vi "Dimmer FG.vi"(7 "Operation":enum16{"Init", "Run", "Close Ref"}(ring)=enum."Run", 8 "error in":errorcluster, 10 "dimmer":i8) -> (0 "error out":errorcluster)   [LabVIEW 2013]
uses:
  System.Management
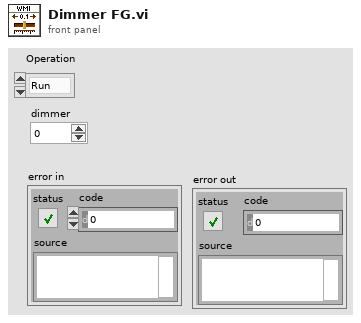
[diagram p1: front panel]
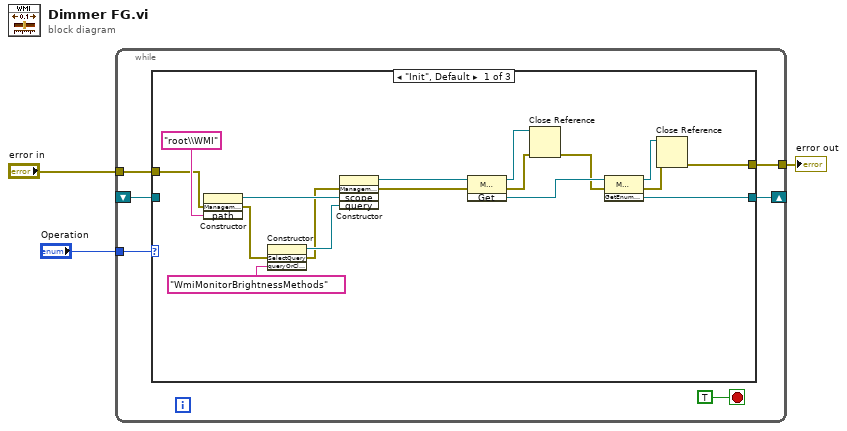
[diagram p0: block diagram]
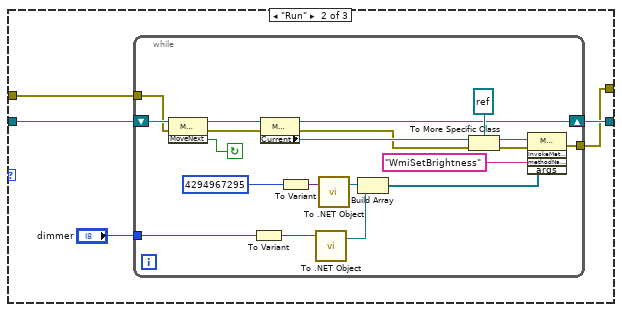
[diagram p2: hidden frame]
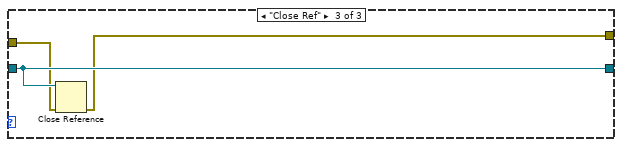
[diagram p3: hidden frame]
diagram:
  n1 = while {
    shift-right: [w9] -> _
    shift-left: _ -> [w8]
    tunnel: "Operation" -> [w6]
    tunnel: "error in" -> [w5]
    tunnel: [w4] -> w1
    stop <- TRUE stop-if-true
    n2 = case shown="\"Init\", Default" w6 {
      tunnel: [w18 w30 w54] -> w9
      tunnel: w8 -> [_ w29 w54]
      tunnel: w5 -> [w16 w28 w53]
      tunnel: [w15 w27 w52] -> w4
      frame "Init", Default {
        n3 = constructor class="ManagementScope"(error in=w16, "path"="root\\WMI") -> (reference out=w22:refnum<k24>, error out=w14:errorcluster)  [unwired: 2 in, 2 out]
        n4 = constructor class="SelectQuery"(error in=w14, "queryOrClassName"="WmiMonitorBrightnessMethods") -> (reference out=w20:refnum<k24>, error out=w13:errorcluster)  [unwired: 2 in, 2 out]
        n5 = constructor class="ManagementObjectSearcher"(error in=w13, "scope"=w22, "query"=w20) -> (reference out=w26:refnum<k24>, error out=w24:errorcluster)  [unwired: 2 in, 3 out]
        n6 = invoke class="ManagementObjectSearcher" method="Get"(reference=w26, error in=w24) -> (reference out=w19:refnum<k24>, error out=w12:errorcluster, "Get"=w25:refnum<k24>)  [unwired: 1 in]
        n7 = Close Reference(reference=w19, error in (no error)=w12) -> (error out=w11:errorcluster)
        n8 = invoke class="ManagementObjectCollection" method="GetEnumerator"(reference=w25, error in=w11) -> (reference out=w17:refnum<k24>, error out=w10:errorcluster, "GetEnumerator"=w18:refnum<k24>)  [unwired: 1 in]
        n9 = Close Reference(reference=w17, error in (no error)=w10) -> (error out=w15:errorcluster)
      }
      frame "Run" {
        n10 = while {
          shift-right: [w43] -> w30
          shift-left: w29 -> [w51]
          tunnel: "dimmer" -> [w34]
          tunnel: w28 -> [w33]
          tunnel: [w32] -> w27
          stop <- w50 continue-if-true
          n11 = invoke class="ManagementObjectCollection+Mana" method="MoveNext"(reference=w51, error in=w33) -> (reference out=w49:refnum<k24>, error out=w48:errorcluster, "MoveNext"=w50:bool)  [unwired: 1 in]
          n12 = To Variant(anything=w34) -> (Variant=w41:variant)
          n13 = property class="ManagementObjectCollection+Mana"(reference=w49, error in=w48) -> (reference out=w43:refnum<k24>, error out=w36:errorcluster, "Current"=w47:refnum<k24>)
          n14 = To Variant(anything=u32 4294967295) -> (Variant=w42:variant)
          n15 = call <vilib>:"To .NET Object.vi"("anything"=w41) -> (".NET object"=w38:refnum<k24>)  [unwired: 1 in, 1 out]
          n16 = call <vilib>:"To .NET Object.vi"("anything"=w42) -> (".NET object"=w39:refnum<k24>)  [unwired: 1 in, 1 out]
          n17 = Build Array(w39, w38) -> (w37:refnum<k24>[])
          n18 = To More Specific Class(target class=refnum<k24> refnum ("Current"), reference=w47, error in=w36) -> (specific class reference=w45:refnum<k24>, error out=w35:errorcluster)
          n19 = invoke class="ManagementObject" method="InvokeMethod"(reference=w45, error in=w35, "methodName"="WmiSetBrightness", "args"=w37) -> (error out=w32:errorcluster)  [unwired: 1 in, 4 out]
        }
      }
      frame "Close Ref" {
        n20 = Close Reference(reference=w54, error in (no error)=w53) -> (error out=w52:errorcluster)
      }
    }
  }
  "error out" <- w1
